vi "Write Hardware.vi"(8 "error in (no error)":errorcluster, 11 "Sensor & Control in":refnum<class "Sensor & Control.lvclass">) -> (0 "error out":errorcluster, 3 "Sensor & Control out":refnum<class "Sensor & Control.lvclass">)   [LabVIEW 2013, in "Sensor & Control.lvlib" / "Sensor & Control.lvclass"]
uses:
  Sensor & Control.lvclass
  <vilib>/Instr/_visa.llb/VISA Flush IO Buffer Mask.ctl
  Sensor & Control.lvclass/Sensor & Control.ctl
  Read VISA.vi
  PluginInterface/PluginInterface.lvlibp/PluginInterfaceClass/Read DVR.vi
  PluginInterface/PluginInterface.lvlibp/PluginInterfaceClass/Read Name.vi
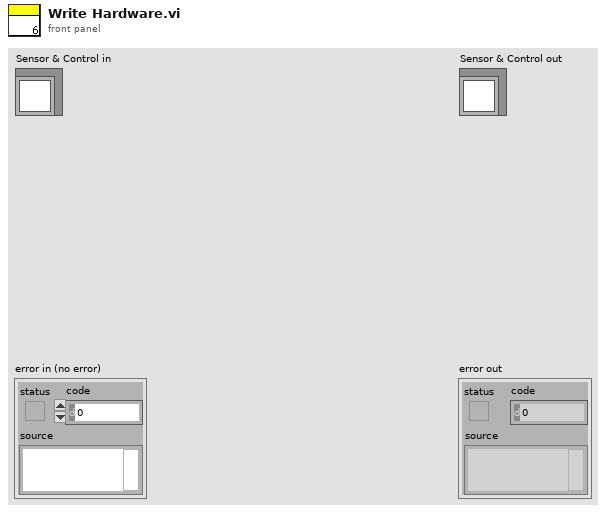
[diagram p1: front panel]
types:
  T1 = typedef "VISA Flush IO Buffer Mask.ctl" = u16
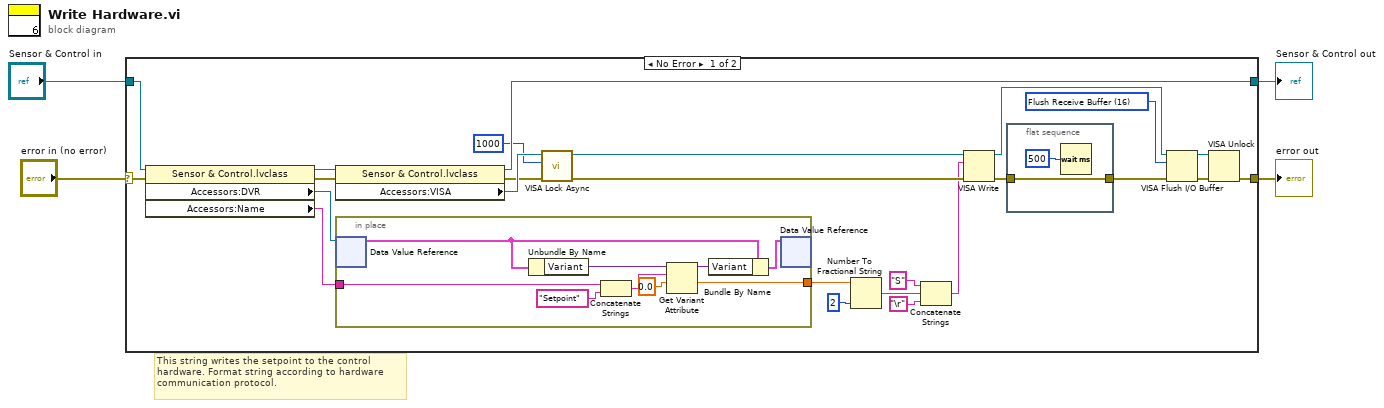
[diagram p0: block diagram]
diagram:
  # "This string writes the setpoint to the control \nhardware. Format string according to hardware\ncommunication protocol."
  n1 = case shown="No Error" "error in (no error)" {
    selector: "error in (no error)" -> [w28 w42]
    tunnel: [w20 w42] -> w1
    tunnel: [w25 w41] -> w2
    tunnel: "Sensor & Control in" -> [w29 w41]
    frame No Error {
      w14 = T1 16 items=["Flush Receive Buffer"=16, "Write Transmit Buffer to Device"=32, "Flush Receive Buffer (No I/O)"=64, "Flush Transmit Buffer"=128] ("Mask")
      n2 = property class="Sensor & Control.lvclass"(reference=w29, error in=w28) -> (reference out=w5:refnum<class "Sensor & Control.lvclass">, error out=w6:errorcluster, "Accessors:DVR"=w27:refnum<data-value>, "Accessors:Name"=w7:string)
      n3 = property class="Sensor & Control.lvclass"(reference=w5, error in=w6) -> (reference out=w25:refnum<class "Sensor & Control.lvclass">, error out=w21:errorcluster, "Accessors:VISA"=w26:refnum<visa-resource-name>)
      n4 = in-place {
        in-place-border: [w35] -> w13
        in-place-border: w7 -> [w33]
        n5 = in-place-dvr #1(w27) -> (w37:cluster{"Array":string[], "Variant":variant})  [unwired: 1 out]
        n6 = Unbundle By Name(w37) -> ("Variant"=w39:variant)
        n7 = Concatenate Strings(w33, "Setpoint") -> (w32:string)
        n8 = Get Variant Attribute(Variant=w39, name=w32, default value (empty Variant)=0.0) -> (duplicate Variant=w38:variant, value=w35:dbl)  [unwired: 1 in, 2 out]
        n9 = Bundle By Name(cluster=w37, "Variant"=w38) -> (w40:cluster{"Array":string[], "Variant":variant})
        n10 = in-place-dvr #1(w40) -> ()  [unwired: 2 out]
      }
      n11 = call <vilib>:"VISA Lock Async.vi"("error in (no error)"=w21, "timeout (0)"=u32 1000, "VISA resource name"=w26) -> ("error out"=w23:errorcluster, "VISA resource name out"=w22:refnum<visa-resource-name>)  [unwired: 6 in, 1 out]
      n12 = Number To Fractional String(number=w13, precision (6)=i16 2) -> (F-format string=w18:string)  [unwired: 2 in]
      n13 = Concatenate Strings("S" ("string"), w18, "\r") -> (w12:string)
      n14 = VISA Write(VISA resource name=w22, write buffer=w12, error in (no error)=w23) -> (VISA resource name out=w11:refnum<visa-resource-name>, error out=w10:errorcluster)  [unwired: 1 out]
      n15 = flat-sequence {
        tunnel: [w30] -> w15
        tunnel: w10 -> [w30]
        frame #0 {
          n16 = Wait (ms)(milliseconds to wait=u32 500) -> ()  [unwired: 1 out]
        }
      }
      n17 = VISA Flush I/O Buffer(VISA resource name=w11, mask (16)=w14, error in (no error)=w15) -> (VISA resource name out=w8:refnum<visa-resource-name>, error out=w9:errorcluster)
      n18 = VISA Unlock(8:w9, 11:w8) -> (0:w20:errorcluster)  [unwired: 1 out]
    }
    frame Error {
    }
  }
  "error out" <- w1
  "Sensor & Control out" <- w2
